vi "ma_Check Block Size no State (CDB).vi"(6 "state info":T2 {"real spectrum" format="%0.2f"; "averages completed" format="%0.2f"; "df" format="%0.2f"; "complex spectrum" format="%0.2f"; "spectrum parameters"."window" items=["Rectangle"=0, "Hanning"=1, "Hamming"=2, "Blackman-Harris"=3, "Exact Blackman"=4, "Blackman"=5, "Flat Top"=6, "4 Term B-Harris "=7, "7 Term B-Harris"=8, "Low Sidelobe"=9, "Blackman Nuttall"=11, "Triangle"=30, "Bartlett-Hanning"=31, "Bohman"=32, "Parzen"=33, "Welch"=34, "Kaiser"=60, "Dolph-Chebyshev"=61, "Gaussian"=62]; "dt" format="%0.2f"; "timestamp" format="%0.2f"; "dt history" format="%0.2f"; "t0 history" format="%0.2f"}, 7 "averaging parameters":T3={"averaging mode"=enum."No averaging", "weighting mode"=enum."Exponential", "number of averages"=10} {"number of averages" min=1}, 8 "error in":errorcluster, 9 "caller VI name":string, 10 "restart averaging (F)":bool, 11 "time signal":waveform(cdb)) -> (0 "error out":errorcluster, 3 "force restart averaging":bool, 4 "state info":T2 {"real spectrum" format="%0.2f"; "averages completed" format="%0.2f"; "df" format="%0.2f"; "complex spectrum" format="%0.2f"; "spectrum parameters"."window" items=["Rectangle"=0, "Hanning"=1, "Hamming"=2, "Blackman-Harris"=3, "Exact Blackman"=4, "Blackman"=5, "Flat Top"=6, "4 Term B-Harris "=7, "7 Term B-Harris"=8, "Low Sidelobe"=9, "Blackman Nuttall"=11, "Triangle"=30, "Bartlett-Hanning"=31, "Bohman"=32, "Parzen"=33, "Welch"=34, "Kaiser"=60, "Dolph-Chebyshev"=61, "Gaussian"=62]; "dt" format="%0.2f"; "timestamp" format="%0.2f"; "dt history" format="%0.2f"; "t0 history" format="%0.2f"})   [LabVIEW 2020, in "NI_MAPro.lvlib"]
uses:
  NI_MAPro.lvlib
  windowTd.ctl
  NI_MABase.lvlib
  NI_AALPro.lvlib
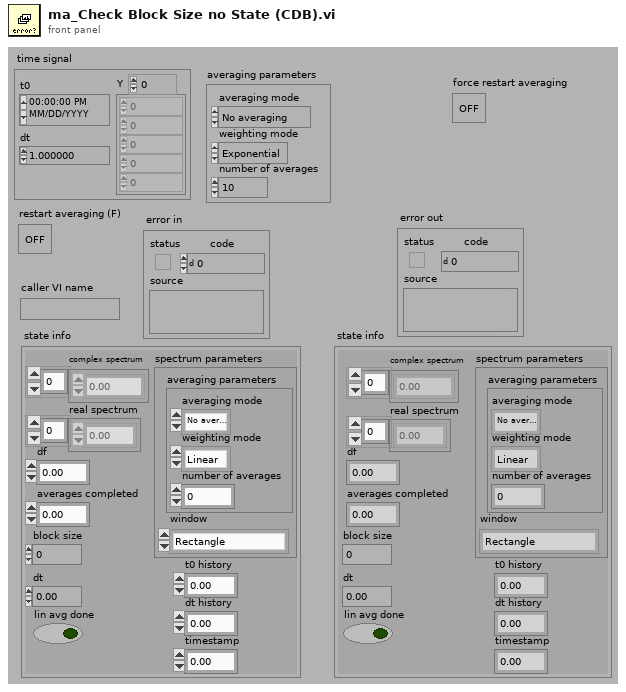
[diagram p1: front panel]
types:
  T1 = typedef "NI_AALPro.lvlib/windowTd.ctl" = u32
  T2 = cluster{"block size":i32, "dt":dbl, "spectrum parameters":cluster{"averaging parameters":cluster{"averaging mode":enum16{"No averaging", "Vector averaging", "RMS averaging", "Peak hold"}, "weighting mode":enum16{"Linear", "Exponential"}, "number of averages":u32}, "window":T1}, "df":dbl, "averages completed":dbl, "complex spectrum":cdb[], "real spectrum":dbl[], "t0 history":dbl, "dt history":dbl, "timestamp":dbl, "lin avg done":bool}
  T3 = cluster{"averaging mode":enum16{"No averaging", "Vector averaging", "RMS averaging", "Peak hold"}, "weighting mode":enum16{"Linear", "Exponential"}, "number of averages":u32}
  T4 = enum16{"No averaging", "Vector averaging", "RMS averaging", "Peak hold"}
  T5 = cluster{"status":bool, "code":i32, "caller VI name":string}
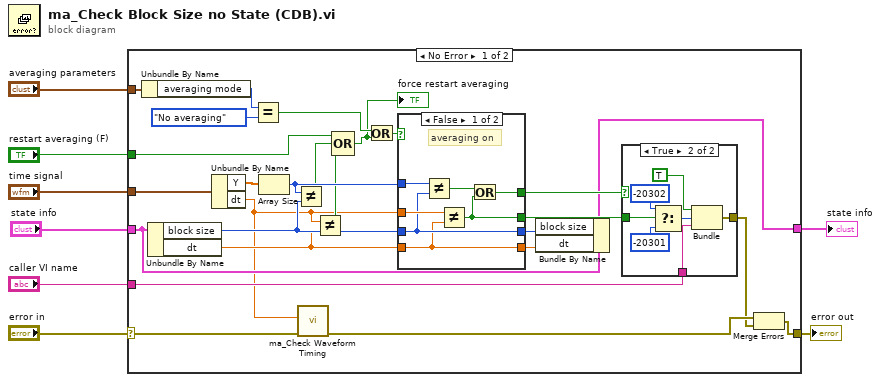
[diagram p0: block diagram]
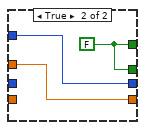
[diagram p2: hidden frame]
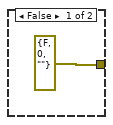
[diagram p3: hidden frame]
diagram:
  n1 = case shown="No Error" "error in" {
    selector: "error in" -> [w13 w53]
    tunnel: [w28 w53] -> w8
    tunnel: "restart averaging (F)" -> [w21 _]
    tunnel: "time signal" -> [w30 _]
    tunnel: "averaging parameters" -> [w29 _]
    tunnel: "caller VI name" -> [w27 _]
    tunnel: "state info" -> [w22 w54]
    tunnel: [w23 w54] -> w1
    frame No Error {
      n2 = Unbundle By Name(w29) -> ("averaging mode"=w32:T4)
      n3 = Unbundle By Name(w22) -> ("block size"=w19:i32, "dt"=w10:dbl)
      n4 = Unbundle By Name(w30) -> ("Y"=w26:cdb[], "dt"=w9:dbl)
      n5 = Equal?(x=w32, y=T4."No averaging" ("averaging mode")) -> (x = y?=w16:bool)
      n6 = Array Size(array=w26) -> (size(s)=w20:i32)
      n7 = Not Equal?(x=w20, y=w19) -> (x != y?=w18:bool)
      n8 = call "ma_Check Waveform Timing.vi"("error in (no error)"=w13, "dt"=w9) -> ("error out"=w12:errorcluster)  [unwired: 1 in, 8 out]
      n9 = Not Equal?(x=w9, y=w10) -> (x != y?=w17:bool)
      n10 = Compound Arithmetic op=OR(w21, w18, w17) -> (w14:bool)
      "force restart averaging" <- w14
      n11 = Or(x=w16, y=w14) -> (x .or. y?=w15:bool)
      n12 = case shown="False" w15 {
        tunnel: w20 -> [w41 w44]
        tunnel: w19 -> [w38 _]
        tunnel: [w38 w44] -> w25
        tunnel: [w37 w43] -> w24
        tunnel: w9 -> [w40 w43]
        tunnel: w10 -> [w37 _]
        tunnel: [w36 w42] -> w34
        tunnel: [w35 w42] -> w31
        frame False {
          # "averaging on"
          n13 = Not Equal?(x=w41, y=w38) -> (x != y?=w39:bool)
          n14 = Not Equal?(x=w40, y=w37) -> (x != y?=w35:bool)
          n15 = Or(x=w39, y=w35) -> (x .or. y?=w36:bool)
        }
        frame True {
          w42 = FALSE
        }
      }
      n16 = Bundle By Name(cluster=w22, "block size"=w25, "dt"=w24) -> (w23:T2)
      n17 = case shown="True" w34 {
        tunnel: [errorcluster {"status"=FALSE, "code"=0, "source"=""} ("error in") w52] -> w11
        tunnel: w31 -> [_ w51]
        tunnel: w27 -> [_ w48]
        frame False {
        }
        frame True {
          n18 = Select(t=-20302 ("code"), s=w51, f=-20301 ("code")) -> (s? t:f=w49:i32)
          n19 = Bundle("status"=TRUE, "code"=w49, "caller VI name"=w48) -> (w52:T5)  [unwired: 1 out]
        }
      }
      n20 = Merge Errors(w12, w11) -> (w28:errorcluster)
    }
    frame Error {
    }
  }
  "error out" <- w8
  "state info" <- w1
